vi "wr_lbne.vi"(1 "DATA":u32 format="%x", 2 "ADDRESS":u16) -> (0 "REG_WR":string)   [LabVIEW 2015]
doc: "This VI is designed to be used with the UDP Receiver VI. Run the UDP Receiver.vi first.\n\nThe UDP protocol differs from TCP in that there is no error-checking with the packets of information that are sent, and thus no guarantee whatsoever that an intended recipient will actually receive a given piece of data.\n\nUDP does offer the ability to \"broadcast\" data across a network--simply specify an IP Address of all ones (255.255.255.255) to attempt to broadcast information network-wide. Keep in mind that routers and other network hardware will generally refuse to forward the broadcast beyond certain points, so the extent of the broadcast will in practice be limited."
uses:
  LBNE_Global .vi
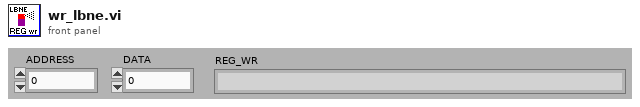
[diagram p1: front panel]
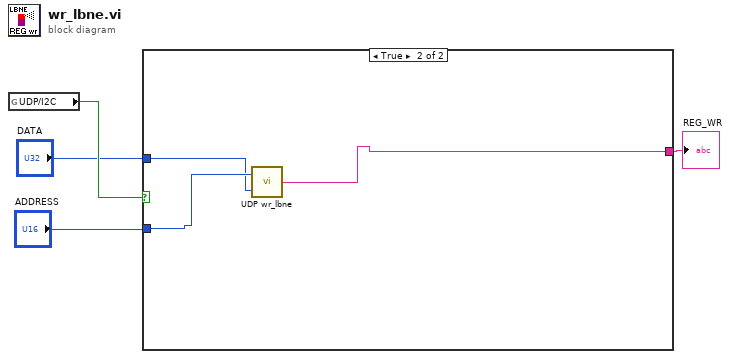
[diagram p0: block diagram]
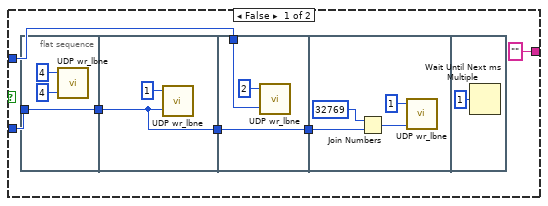
[diagram p2: hidden frame]
diagram:
  n1 = global read "LBNE_Global .vi" "UDP/I2C"() -> (w4:bool)
  n2 = case shown="True" w4 {
    tunnel: "DATA" -> [w8 w24]
    tunnel: "ADDRESS" -> [w9 w25]
    tunnel: ["" ("REG_WR") w26] -> w2
    frame False {
      n3 = flat-sequence {
        tunnel: w9 -> [w13]
        tunnel: [w13] -> w5
        tunnel: [w14] -> w7
        tunnel: w5 -> [w14]
        tunnel: w8 -> [w17]
        tunnel: w7 -> [w16]
        tunnel: [w16] -> w6
        tunnel: w6 -> [w21]
        frame #0 {
          n4 = call "UDP wr_lbne.vi"("DATA"=u32 4, "ADDRESS"=u16 4) -> ()  [unwired: 1 out]
        }
        frame #1 {
          n5 = call "UDP wr_lbne.vi"("DATA"=w14, "ADDRESS"=u16 1) -> ()  [unwired: 1 out]
        }
        frame #2 {
          n6 = call "UDP wr_lbne.vi"("DATA"=w17, "ADDRESS"=u16 2) -> ()  [unwired: 1 out]
        }
        frame #3 {
          n7 = Join Numbers(hi=u16 32769, lo=w21) -> ((hi.lo)=w19:u32)
          n8 = call "UDP wr_lbne.vi"("DATA"=w19, "ADDRESS"=u16 1) -> ()  [unwired: 1 out]
        }
        frame #4 {
          n9 = Wait Until Next ms Multiple(millisecond multiple=u32 1) -> ()  [unwired: 1 out]
        }
      }
    }
    frame True {
      n10 = call "UDP wr_lbne.vi"("DATA"=w24, "ADDRESS"=w25) -> ("REG_WR"=w26:string)
    }
  }
  "REG_WR" <- w2
